vi "next state.vi"(8 "error in (no error)":errorcluster, 11 "Data in":T1={"link 1 angle"=0.0, "link 2 angle"=0.0, "link 1 length"=0.0, "link 2 length"=0.0, "Current arm location"=[{"X"=0.0, "Y"=0.0}, {"X"=-37.249783598972314, "Y"=33.353464914904016}, {"X"=-74.49956719794463, "Y"=66.70692982980803}], "Link Picture"=bytes[1162], "Desired Location"={"Desired X"=0.0, "Desired Y"=0.0}, "Next Location"={"Next X"=0.0, "Next Y"=0.0}, "Error"={"Joint1 error"=0.0, "Joint2 error"=0.0}, "tdms data"=refnum, "de/dt"={"joint1 de/dt"=0.0, "joint2 de/dt"=0.0}, "Voltages"={"Joint1 voltage"=0.0, "Joint2 voltage"=0.0}, "Time"=0.0, "dt"=0.0, "counts/rev"=0.0, "kp"=0.0, "kd"=0.0, "ki"=0.0, "Int(error)"={"joint1 int(e)"=0.0, "joint2 int(e)"=0.0}, "Desired angles"={"theta 1"=0.0, "theta 2"=0.0}, "Current counts"={"theta 1"=0.0, "theta 2"=0.0}, "Desired Counts"={"theta 1"=0.0, "theta 2"=0.0}, "Preivous Error"={"Joint1 Previous error"=0.0, "Joint2 Previous error"=0.0}, "Counts/s"=0.0, "Correct counter"=0}) -> (0 "error out":errorcluster, 2 "Next State":string, 3 "Data out":T1={"link 1 angle"=0.0, "link 2 angle"=0.0, "link 1 length"=0.0, "link 2 length"=0.0, "Current arm location"=[{"X"=0.0, "Y"=0.0}, {"X"=-37.249783598972314, "Y"=33.353464914904016}, {"X"=-74.49956719794463, "Y"=66.70692982980803}], "Link Picture"=bytes[1162], "Desired Location"={"Desired X"=0.0, "Desired Y"=0.0}, "Next Location"={"Next X"=0.0, "Next Y"=0.0}, "Error"={"Joint1 error"=0.0, "Joint2 error"=0.0}, "tdms data"=refnum, "de/dt"={"joint1 de/dt"=0.0, "joint2 de/dt"=0.0}, "Voltages"={"Joint1 voltage"=0.0, "Joint2 voltage"=0.0}, "Time"=0.0, "dt"=0.0, "counts/rev"=0.0, "kp"=0.0, "kd"=0.0, "ki"=0.0, "Int(error)"={"joint1 int(e)"=0.0, "joint2 int(e)"=0.0}, "Desired angles"={"theta 1"=0.0, "theta 2"=0.0}, "Current counts"={"theta 1"=0.0, "theta 2"=0.0}, "Desired Counts"={"theta 1"=0.0, "theta 2"=0.0}, "Preivous Error"={"Joint1 Previous error"=0.0, "Joint2 Previous error"=0.0}, "Counts/s"=0.0, "Correct counter"=0})   [LabVIEW 2017]
uses:
  Type Defs/Host Data.ctl
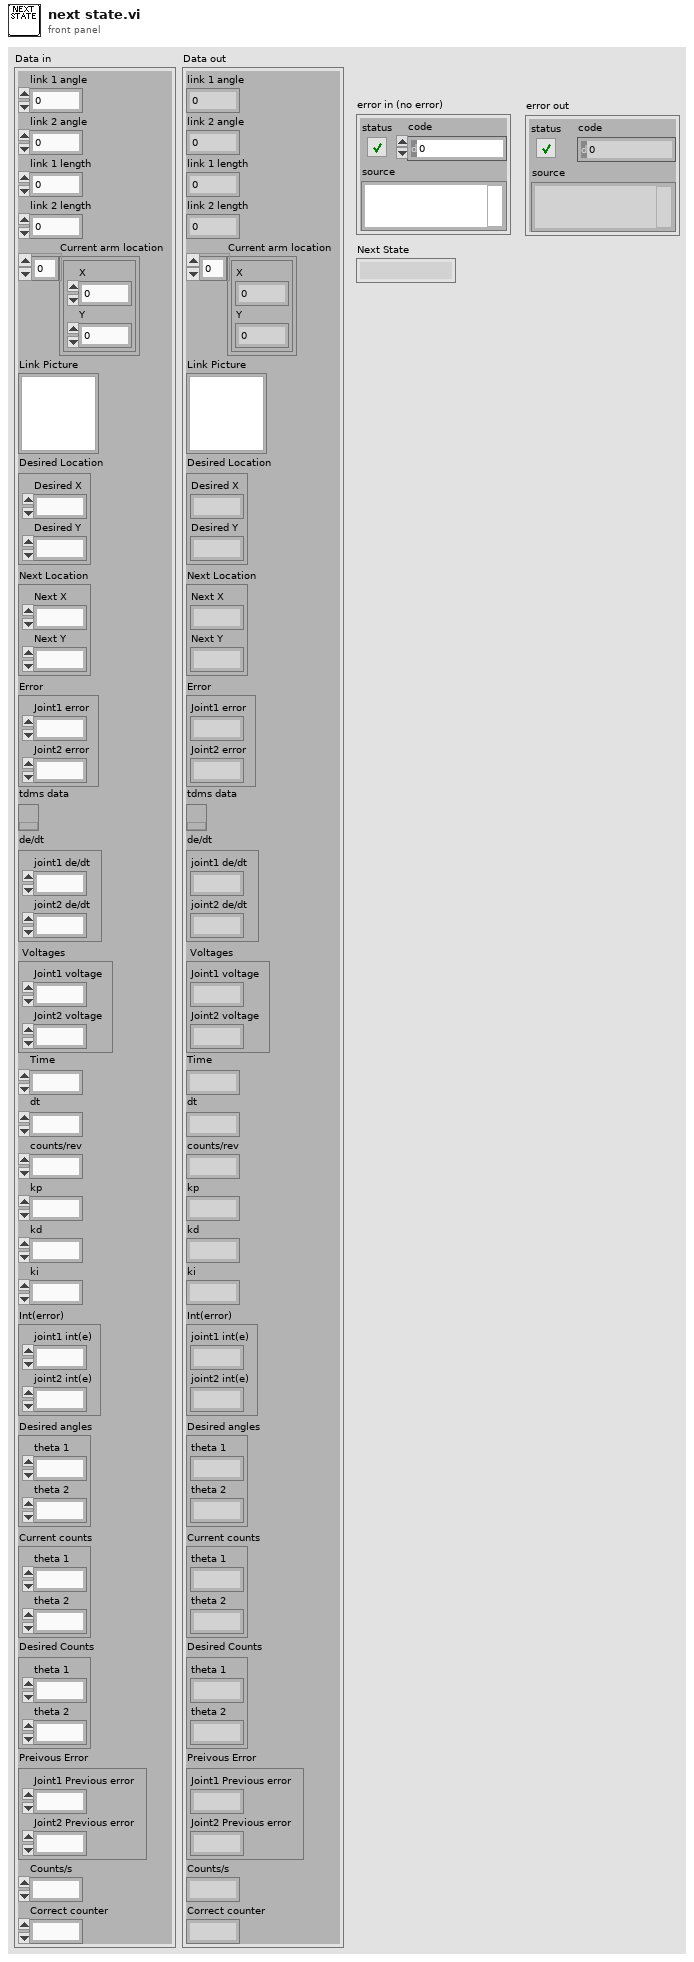
[diagram p1: front panel]
types:
  T1 = typedef "Host Data.ctl" = cluster{"link 1 angle":dbl, "link 2 angle":dbl, "link 1 length":dbl, "link 2 length":dbl, "Current arm location":cluster{"X":dbl, "Y":dbl}[], "Link Picture":picture, "Desired Location":cluster{"Desired X":dbl, "Desired Y":dbl}, "Next Location":cluster{"Next X":dbl, "Next Y":dbl}, "Error":cluster{"Joint1 error":dbl, "Joint2 error":dbl}, "tdms data":refnum<k34>, "de/dt":cluster{"joint1 de/dt":dbl, "joint2 de/dt":dbl}, "Voltages":cluster{"Joint1 voltage":dbl, "Joint2 voltage":dbl}, "Time":dbl, "dt":dbl, "counts/rev":dbl, "kp":dbl, "kd":dbl, "ki":dbl, "Int(error)":cluster{"joint1 int(e)":dbl, "joint2 int(e)":dbl}, "Desired angles":cluster{"theta 1":dbl, "theta 2":dbl}, "Current counts":cluster{"theta 1":dbl, "theta 2":dbl}, "Desired Counts":cluster{"theta 1":dbl, "theta 2":dbl}, "Preivous Error":cluster{"Joint1 Previous error":dbl, "Joint2 Previous error":dbl}, "Counts/s":dbl, "Correct counter":i32}
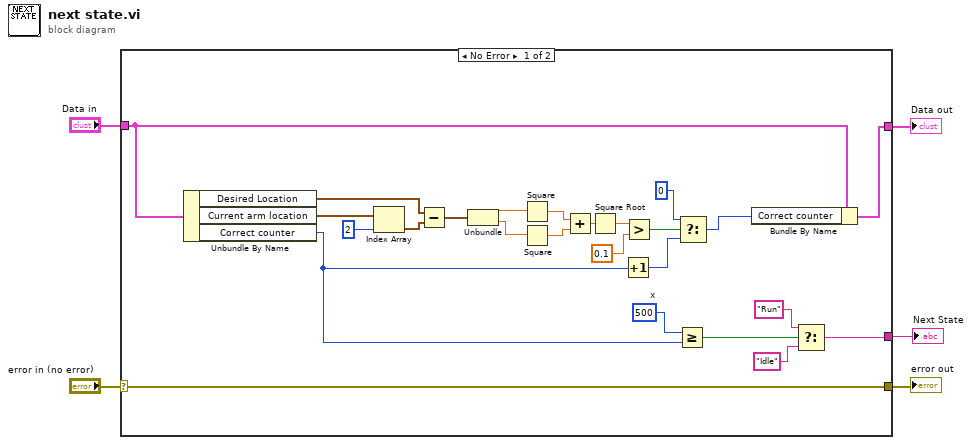
[diagram p0: block diagram]
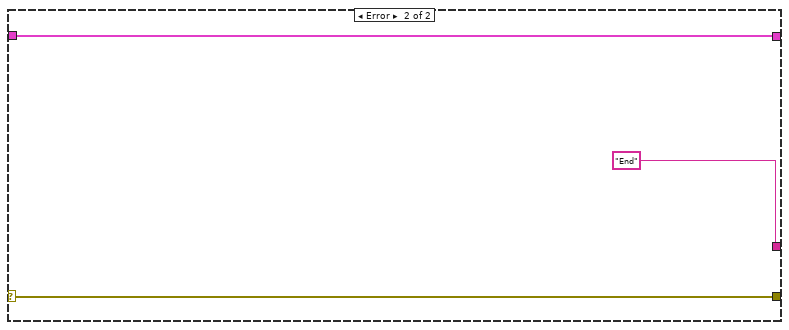
[diagram p2: hidden frame]
diagram:
  n1 = case shown="No Error" "error in (no error)" {
    selector: "error in (no error)" -> [w26 w32]
    tunnel: "Data in" -> [w14 w33]
    tunnel: [w13 w33] -> w3
    tunnel: [w26 w32] -> w2
    tunnel: [w15 "End"] -> w1
    frame No Error {
      w6 = 500  # x
      n2 = Unbundle By Name(w14) -> ("Desired Location"=w28:cluster{"Desired X":dbl, "Desired Y":dbl}, "Current arm location"=w30:cluster{"X":dbl, "Y":dbl}[], "Correct counter"=w7:i32)
      n3 = Index Array(array=w30, index=2) -> (element=w27:cluster{"X":dbl, "Y":dbl})
      n4 = Subtract(x=w28, y=w27) -> (x-y=w25:cluster{dbl, dbl})
      n5 = Unbundle(w25) -> (w24:dbl, w23:dbl)
      n6 = Square(x=w24) -> (x^2=w21:dbl)
      n7 = Square(x=w23) -> (x^2=w22:dbl)
      n8 = Add(x=w21, y=w22) -> (x+y=w20:dbl)
      n9 = Square Root(x=w20) -> (sqrt(x)=w19:dbl)
      n10 = Increment(x=w7) -> (x+1=w9:i32)
      n11 = Greater?(x=w19, y=0.1) -> (0:w12:bool)
      n12 = Greater Or Equal?(x=w6, y=w7) -> (x >= y?=w8:bool)
      n13 = Select(t=0, s=w12, f=w9) -> (s? t:f=w11:i32)
      n14 = Bundle By Name(cluster=w14, "Correct counter"=w11) -> (w13:T1)
      n15 = Select(t="Run", s=w8, f="Idle") -> (s? t:f=w15:string)
    }
    frame Error {
    }
  }
  "Data out" <- w3
  "error out" <- w2
  "Next State" <- w1
